vi "FTW-ProjectItem-Tag-Enumerate.vi"(0 "ProjectItem":refnum<vi>, 5 "Tag Name Regex Filter (blank returns all tags)":string, 11 "error in":errorcluster) -> (4 "ProjectItem out":refnum<vi>, 6 "Matching Tags":string[](array[string]), 8 "Regex Results":cluster{"Match":string, "Submatches":string[]}[](array[cluster]), 15 "error out":errorcluster)   [LabVIEW 2012]
panel:
  # "Inputs"
  # "Outputs"
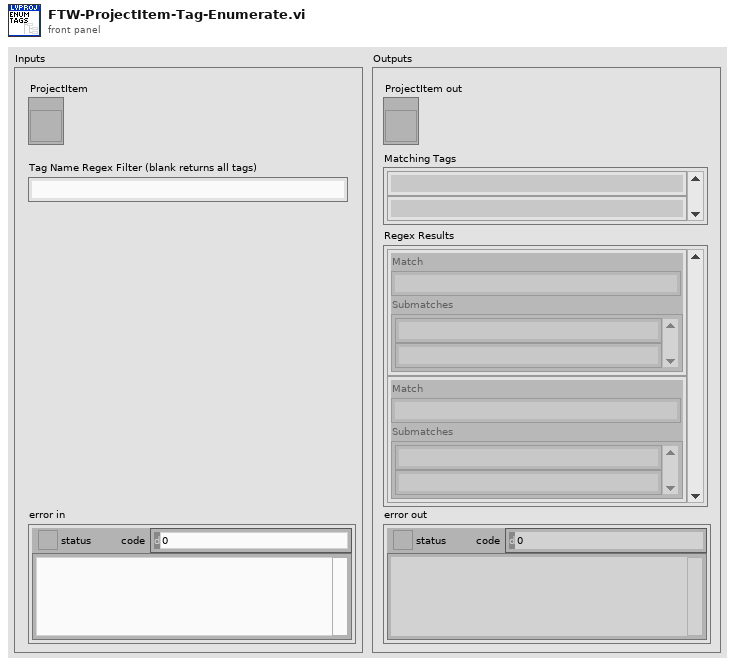
[diagram p1: front panel]
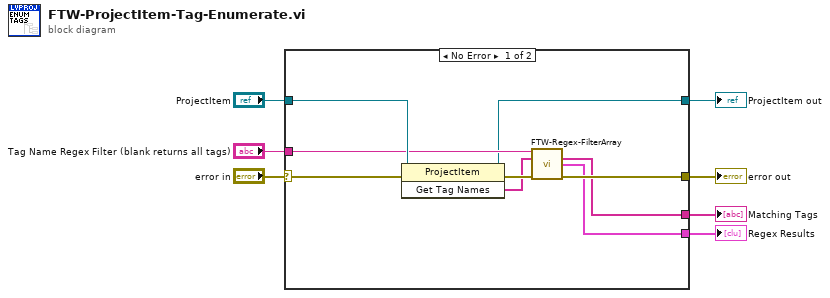
[diagram p0: block diagram]
diagram:
  n1 = case shown="No Error" "error in" {
    selector: "error in" -> [w16 w18]
    tunnel: [w13 w18] -> w7
    tunnel: "Tag Name Regex Filter (blank returns all tags)" -> [w11 _]
    tunnel: [w10 _] -> w4
    tunnel: "ProjectItem" -> [w15 w17]
    tunnel: [w9 w17] -> w2
    tunnel: [w8 _] -> w1
    frame No Error {
      n2 = invoke class="ProjectItem" method="Get Tag Names"(reference=w15, error in=w16) -> (reference out=w9:refnum<vi>, error out=w14:errorcluster, "Get Tag Names"=w12:string[])  [unwired: 1 in]
      n3 = call "FTW-Regex-FilterArray.vi"("Regex Filter"=w11, "Input Array"=w12, "error in"=w14) -> ("Matching Items"=w10:string[], "Regex Results"=w8:cluster{"Match":string, "Submatches":string[]}[], "error out"=w13:errorcluster)  [unwired: 10 in]
    }
    frame Error {
    }
  }
  "error out" <- w7
  "Matching Tags" <- w4
  "ProjectItem out" <- w2
  "Regex Results" <- w1
